vi "子VI-配置信息显示.vi"(9 "视频检测帧间隔output":i8, 10 "是否使用GPU计算output":i8, 11 "模式选择output":i8) -> (2 "配置信息说明":string)   [LabVIEW 2018]
panel:
  out "标尺.范围:最大值":dbl
  out "GPU":string="使用GPU"
  out "导入配置":u8(slide) scale=0.0..8.0
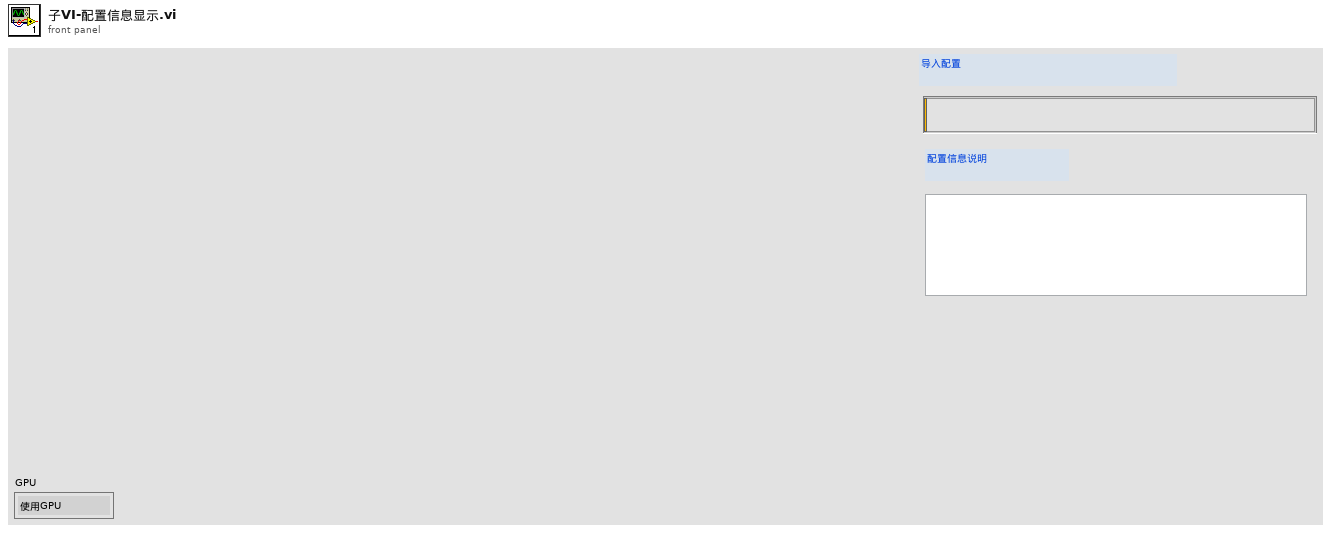
[diagram p1: front panel]
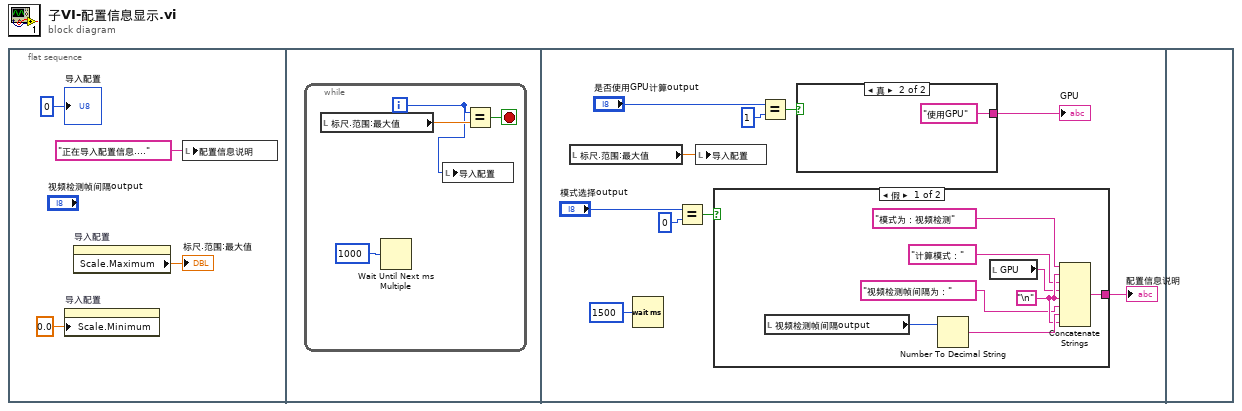
[diagram p0: block diagram]
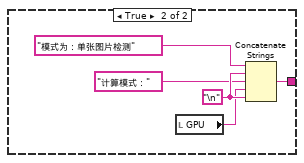
[diagram p2: hidden frame]
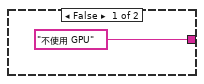
[diagram p3: hidden frame]
diagram:
  n1 = flat-sequence {
    frame #0 {
      n2 = property on="导入配置" class="Slide (严格)"("Scale.Minimum"=0.0 ("标尺.范围:最小值")) -> ()  [unwired: 2 in, 2 out]
      n3 = property on="导入配置" class="Slide (严格)"() -> ("Scale.Maximum"=→"标尺.范围:最大值":dbl)  [unwired: 2 in, 2 out]
      n4 = local write "配置信息说明"("正在导入配置信息...." ("配置信息说明")) -> ()
      "导入配置" <- u8 0 ("导入配置")
    }
    frame #1 {
      n5 = while {
        i -> [w5]
        stop <- w7 stop-if-true
        n6 = local read "标尺.范围:最大值"() -> (w8:dbl)
        n7 = Wait Until Next ms Multiple(millisecond multiple=u32 1000 ("毫秒倍数")) -> ()  [unwired: 1 out]
        n8 = local write "导入配置"(w5) -> ()
        n9 = Equal?(x=w5, y=w8) -> (x = y?=w7:bool)
      }
    }
    frame #2 {
      n10 = local read "标尺.范围:最大值"() -> (w9:dbl)
      n11 = Wait (ms)(milliseconds to wait=u32 1500 ("等待时间（毫秒）")) -> ()  [unwired: 1 out]
      n12 = Equal?(x="模式选择output", y=i8 0) -> (x = y?=w15:bool)
      n13 = local write "导入配置"(w9) -> ()
      n14 = case shown="假" w15 {
        tunnel: [w19 w27] -> w16
        frame False {
          w24 = "\n"
          n15 = local read "视频检测帧间隔output"() -> (w20:i8)
          n16 = Number To Decimal String(number=w20) -> (decimal integer string=w26:string)  [unwired: 1 in]
          n17 = local read "GPU"() -> (w22:string)
          n18 = Concatenate Strings("模式为：视频检测" ("字符串"), w24, "计算模式：" ("字符串"), w22, w24, "视频检测帧间隔为：" ("字符串"), w26, w24) -> (w19:string)
        }
        frame True {
          w31 = "\n"
          n19 = local read "GPU"() -> (w28:string)
          n20 = Concatenate Strings("模式为：单张图片检测" ("字符串"), w31, "计算模式：" ("字符串"), w28, w31) -> (w27:string)
        }
      }
      "配置信息说明" <- w16
      n21 = Equal?(x="是否使用GPU计算output", y=i8 1) -> (x = y?=w13:bool)
      n22 = case shown="真" w13 {
        tunnel: ["不使用 GPU" "使用GPU"] -> w14
        frame False {
        }
        frame True {
        }
      }
      "GPU" <- w14
    }
    frame #3 {
    }
  }
